vi "Configure Timing.vi"(8 "error in (no error)":errorcluster, 10 "Params":variant, 11 "NI DAQmx Base in":refnum<class "NI DAQmx Base.lvclass">) -> (0 "error out":errorcluster, 3 "NI DAQmx Base out":refnum<class "NI DAQmx Base.lvclass">)   [LabVIEW 2020, in "NI DAQmx.lvlib" / "NI DAQmx Base.lvclass"]
uses:
  NI DAQmx Base.lvclass
  NI Analog Output/TypeDefs/Timing Config.ctl
  <vilib>/DAQmx/configure/timing.llb/DAQmx Timing (Sample Clock).vi
  NI DAQmx Base.lvclass/NI DAQmx Base.ctl
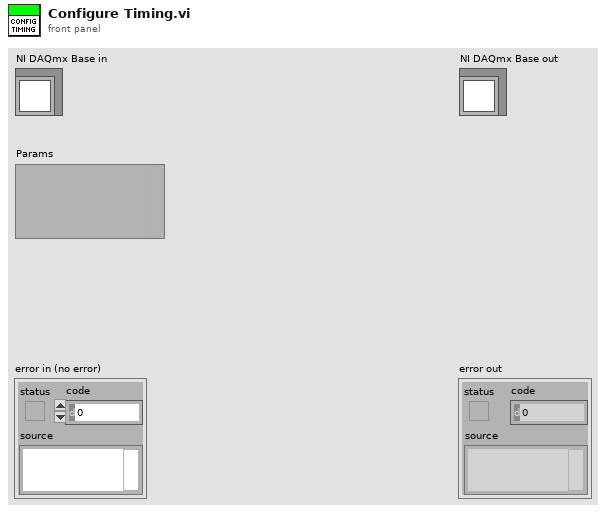
[diagram p1: front panel]
types:
  T1 = typedef "Timing Config.ctl" = cluster{"sample mode":i32, "samples per channel":i32, "rate":dbl, "source":string, "active edge":i32}
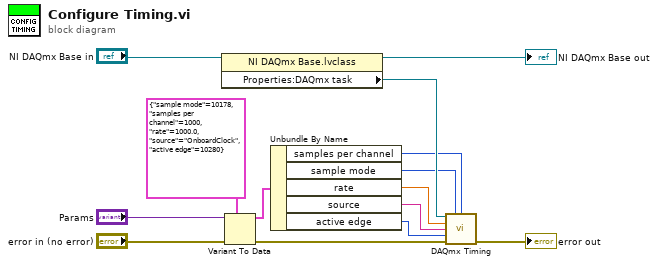
[diagram p0: block diagram]
diagram:
  n1 = property class="NI DAQmx Base.lvclass"(reference="NI DAQmx Base in") -> (reference out=→"NI DAQmx Base out":refnum<class "NI DAQmx Base.lvclass">, "Properties:DAQmx task"=w13:refnum<k21>)  [unwired: 1 in, 1 out]
  n2 = Variant To Data(error in="error in (no error)", type=T1 {"sample mode"=10178, "samples per channel"=1000, "rate"=1000.0, "source"="OnboardClock", "active edge"=10280}, Variant="Params") -> (data=w11:T1, error out=w14:errorcluster)
  n3 = Unbundle By Name(w11) -> ("samples per channel"=w6:i32, "sample mode"=w7:i32, "rate"=w10:dbl, "source"=w9:string, "active edge"=w8:i32)
  n4 = call-poly <vilib>:"DAQmx Timing.vi"("task/channels in"=w13, "sample mode"=w7, "samples per channel"=w6, "rate"=w10, "source"=w9, "active edge"=w8, "error in"=w14) -> ("error out"=→"error out":errorcluster)  [unwired: 7 in, 1 out]
